vi "Activate.vi"(8 "error in (no error)":errorcluster, 11 "Object ref in":T1) -> (0 "error out":errorcluster, 3 "Object ref out":T1)   [LabVIEW 2013, in "HardwareCharacterization.lvlib" / "HC-Main.lvclass"]
uses:
  HC-Main.lvclass
  Object-reference.ctl
  HC-Main.lvclass/HC-Main.ctl
  Application-status.ctl
  UI/Control-names.ctl
  Process1-actions.ctl
  Read UI.vi
  Read Status.vi
  UI/Set-control-enable-multiple.vi
  UI/Set-control-enable-single.vi
  UI/HC-UI.lvclass
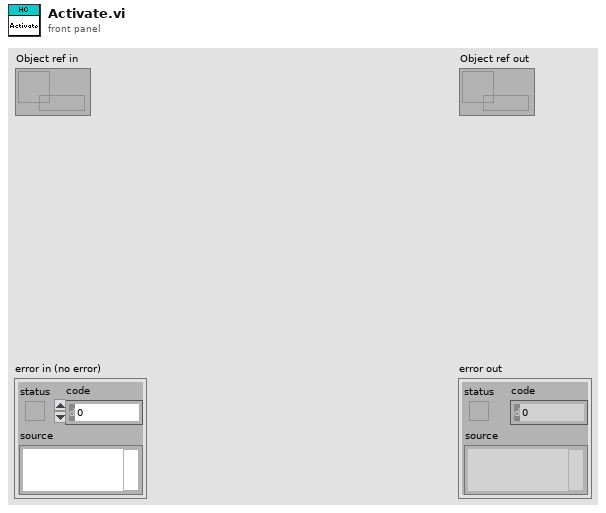
[diagram p1: front panel]
types:
  T1 = typedef "HardwareCharacterization.lvlib/HC-Main.lvclass/Object-reference.ctl" = refnum<data-value>
  T2 = typedef "HardwareCharacterization.lvlib/HC-Main.lvclass/Process1-actions.ctl" = enum16{"Idle", "Activate", "Analyse scan file", "Convert SM1000positions", "Measure SM1000 timings", "Measure laser timings", "Stop", "Abort", "Exit"}
  T3 = typedef "HardwareCharacterization.lvlib/HC-UI.lvclass/Control-names.ctl" = enum16{"Help", "Status", "Load configuration", "Save configuration", "Activate", "Start", "Stop", "Options"}
  T4 = typedef "HardwareCharacterization.lvlib/HC-Main.lvclass/Application-status.ctl" = enum16{"Idle", "Initialized", "Configured", "Activated", "Started", "Paused", "Stopped", "Reset", "Error", "Exited"}
  T5 = typedef "HardwareCharacterization.lvlib/HC-UI.lvclass/Panes-reference.ctl" = refnum<data-value>
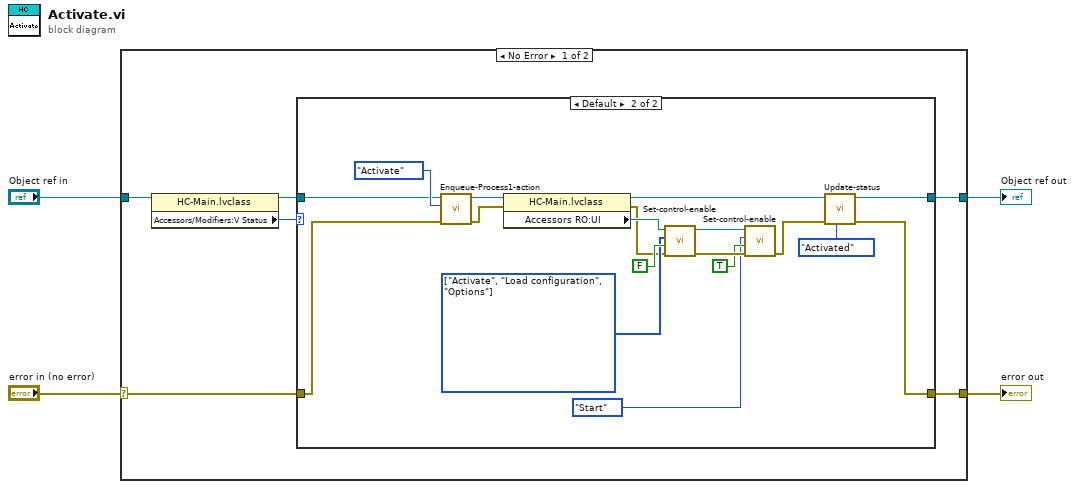
[diagram p0: block diagram]
diagram:
  n1 = case shown="No Error" "error in (no error)" {
    selector: "error in (no error)" -> [w7 w32]
    tunnel: [w10 w32] -> w3
    tunnel: [w9 w31] -> w1
    tunnel: "Object ref in" -> [w8 w31]
    frame No Error {
      n2 = property class="HC-Main.lvclass"(reference=w8) -> (reference out=w6:T1, "Accessors/Modifiers:V Status"=w5:T4)  [unwired: 1 in, 1 out]
      n3 = case shown="Default" w5 {
        tunnel: [w11 w29] -> w10
        tunnel: [w12 w28] -> w9
        tunnel: w7 -> [w11 w13]
        tunnel: w6 -> [w12 w14]
        frame "Initialized", "Started", "Paused" {
        }
        frame Default {
          w24 = T3[] [enum."Activate", enum."Load configuration", enum."Options"] items=["Help", "Status", "Load configuration", "Save configuration", "Activate", "Start", "Stop", "Options"] ("Control names")
          n4 = call "Enqueue-Process1-action.vi"("error in (no error)"=w13, "Action"=Process1-actions."Activate", "State queue in"=w14) -> ("error out"=w17:errorcluster, "State queue out"=w15:T1)  [unwired: 6 in, 1 out]
          n5 = property class="HC-Main.lvclass"(reference=w15, error in=w17) -> (reference out=w27:T1, error out=w23:errorcluster, "Accessors RO:UI"=w25:T5)
          n6 = call-poly "Set-control-enable.vi"("error in (no error)"=w23, "Enable?"=FALSE, "Control names"=w24, "Panes in"=w25) -> ("error out"=w21:errorcluster, "Panes out"=w22:T5)  [unwired: 6 in]
          n7 = call-poly "Set-control-enable.vi"("error in (no error)"=w21, "Enable?"=TRUE, "Control name"=Control-names."Start", "Panes in"=w22) -> ("error out"=w18:errorcluster)  [unwired: 6 in, 1 out]
          n8 = call "Update-status.vi"("Status"=Application-status."Activated", "error in (no error)"=w18, "Object ref in"=w27) -> ("error out"=w29:errorcluster, "Object ref out"=w28:T1)  [unwired: 7 in]
        }
      }
    }
    frame Error {
    }
  }
  "error out" <- w3
  "Object ref out" <- w1
